vi "Wrap FTQF.vi"(8 "error in (no error)":errorcluster, 11 "VISA resource name":refnum<visa-resource-name>) -> (0 "error out":errorcluster, 3 "VISA resource name out":refnum<visa-resource-name>)   [LabVIEW 2020]
uses:
  support/Serial - Settings.ctl
  <vilib>/Instr/_visa.llb/VISA Configure Serial Port (Instr).vi
panel:
  in  "Select LO Freq. GHz":T1(ring)
  in  "Serial Settings":T2={"baud rate"=2000000, "data bits"=8, "parity"=enum."None", "stop bits"=10, "flow control"=1} {"flow control" items=["None"=0, "XON/XOFF"=1, "RTS/CTS"=2, "DTR/DSR"=4]; "stop bits" items=["1.0"=10, "1.5"=15, "2.0"=20]; "data bits" min=5 max=8 step=1; "baud rate" items=["75"=75, "110"=110, "134"=134, "150"=150, "300"=300, "600"=600, "1200"=1200, "1800"=1800, "2400"=2400, "4800"=4800, "7200"=7200, "9600"=9600, "14400"=14400, "19200"=19200, "28800"=28800, "38400"=38400, "56000"=56000, "57600"=57600, "115200"=115200, "128000"=128000, "230400"=230400]}
  out "Response":string
  out "Frequency GHz":string
  # "2.5, 3.5, 4.5 ... 17.3, 17.4, 17.5"
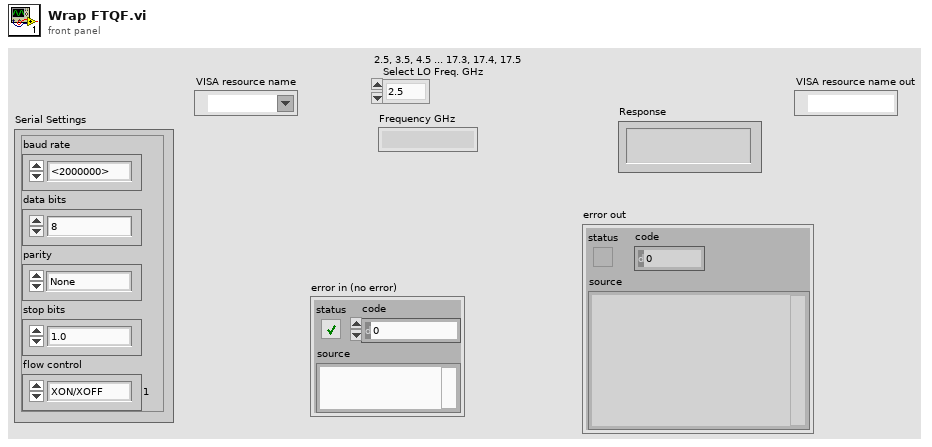
[diagram p1: front panel]
types:
  T1 = enum16{"2.5", "3.5", "4.5", "5.5", "6.5", "7.5", "8.5", "9.5", "10.5", "11.5", "12.5", "13.5", "14.5", "15.5", "16.5", "17.5"}
  T2 = typedef "Serial - Settings.ctl" = cluster{"baud rate":u32, "data bits":u16, "parity":enum16{"None", "Odd", "Even", "Mark", "Space"}, "stop bits":u16, "flow control":u16}
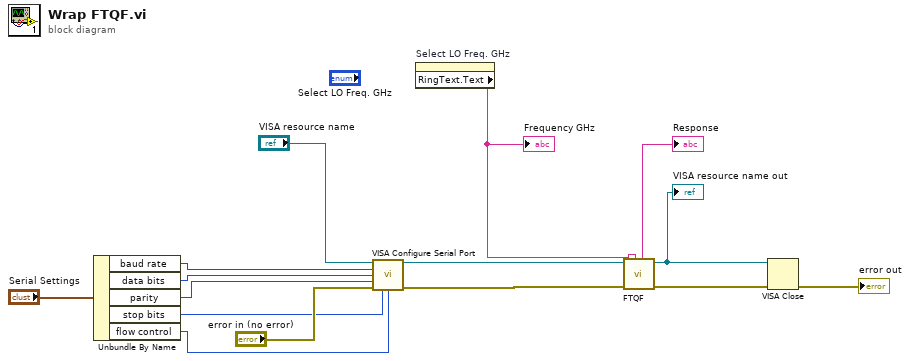
[diagram p0: block diagram]
diagram:
  n1 = Unbundle By Name("Serial Settings") -> ("baud rate"=w6:u32, "data bits"=w5:u16, "parity"=w4:enum16{"None", "Odd", "Even", "Mark", "Space"}, "stop bits"=w3:u16, "flow control"=w2:u16)
  n2 = call-poly "VISA Configure Serial Port"("VISA resource name"="VISA resource name", "baud rate (9600)"=w6, "data bits (8)"=w5, "parity (0:none)"=w4, "error in (no error)"="error in (no error)", "stop bits (10: 1 bit)"=w3, "flow control (0:none)"=w2) -> ("VISA resource name out"=w13:refnum<visa-resource-name>, "error out"=w14:errorcluster)  [unwired: 7 in]
  n3 = property on="Select LO Freq. GHz" class="Enum (strict)"() -> ("RingText.Text"=w1:string)  [unwired: 2 in, 2 out]
  "Frequency GHz" <- w1
  n4 = call "FTQF.vi"("Frequency GHz"=w1, "error in (no error)"=w14, "VISA resource name"=w13) -> ("error out"=w11:errorcluster, "VISA resource name out"=w12:refnum<visa-resource-name>, "Response"=→"Response":string)  [unwired: 6 in]
  "VISA resource name out" <- w12
  n5 = VISA Close(VISA resource name=w12, error in (no error)=w11) -> (error out=→"error out":errorcluster)
